vi "DNP3_Outstation_Main.vi"() -> ()   [LabVIEW 2016, in "DNP3_Outstation_Template.lvlib"]
uses:
  DNP3_Outstation_Template.lvlib
panel:
  out "STOP IND":bool
  out "RESET OS IND":bool
  out "ENABLE OS IND":bool=TRUE
  in  "STOP":bool
  out "MS POLLING? IND":bool=TRUE
  in  "OS Presets":T1(tab)
  in  "Network Settings 1":T2={"port (20000)"=18000, "Master IP"="48.26.87.212", "Master Address"=12345, "Outstation Address "=54321, " update rate"=50}
  in  "DNP3 DataMap 1":T3={"Binary Output Points"=1, "Binary Input Points"=0, "Analog Output Points"=7, "Analog Input Points"=6}
  in  "Settings Cluster":T4={"Default Variation:Analog Input Event (OBJ32)"=1, "Default Variation:Analog Input (OBJ30)"=1, "Default Variation:Binary Input (OBJ01)"=1, "Default Variation:Analog Output (OBJ40)"=4, "Default Variation:Binary Output Event (OBJ11)"=1, "Default Variation:Binary Output (OBJ10)"=1, "Default Variation:Analog Output Event (OBJ42)"=8, "Unsolicited Response Allowed"=FALSE, "Control:Select Timeout (ms)"=0, "Misc:Appl Confirmation Timeout"=0} {"Default Variation:Analog Output Event (OBJ42)" items=["32-bit without Time"=1, "16-bit without Time"=2, "32-bit with Time"=3, "16-bit with Time"=4, "Single-prec without Time"=5, "Double-prec without Time"=6, "Single-prec with Time"=7, "Double-prec with Time"=8]; "Default Variation:Binary Output (OBJ10)" items=["Packed Format"=1, "Output Status with Flags"=2]; "Default Variation:Binary Output Event (OBJ11)" items=["Status without Time"=1, "Status with Time"=2]; "Default Variation:Analog Output (OBJ40)" items=["32-bit with Flag"=1, "16-bit with Flag"=2, "Single-prec with Flag"=3, "Double-prec with Flag"=4]; "Default Variation:Binary Input (OBJ01)" items=["Packed Format"=1, "With Flags"=2]; "Default Variation:Analog Input (OBJ30)" items=["32-bit with Flag"=1, "16-bit with Flag"=2, "32-bit without Flag"=3, "16-bit without Flag"=4, "Single-prec with Flag"=5, "Double-prec with Flag"=6]; "Default Variation:Analog Input Event (OBJ32)" items=["32-bit without Time"=1, "16-bit without Time"=2, "32-bit with Time"=3, "16-bit with Time"=4, "Single-prec without Time"=5, "Double-prec without Time"=6, "Single-prec with Time"=7, "Double-prec with Time"=8]}
  in  "Network Settings 2":T2
  in  "DNP3 DataMap 2":T3
  in  "Settings Cluster 2":T4={"Default Variation:Analog Input Event (OBJ32)"=1, "Default Variation:Analog Input (OBJ30)"=1, "Default Variation:Binary Input (OBJ01)"=1, "Default Variation:Analog Output (OBJ40)"=1, "Default Variation:Binary Output Event (OBJ11)"=1, "Default Variation:Binary Output (OBJ10)"=1, "Default Variation:Analog Output Event (OBJ42)"=1, "Unsolicited Response Allowed"=FALSE, "Control:Select Timeout (ms)"=0, "Misc:Appl Confirmation Timeout"=0} {"Default Variation:Analog Output Event (OBJ42)" items=["32-bit without Time"=1, "16-bit without Time"=2, "32-bit with Time"=3, "16-bit with Time"=4, "Single-prec without Time"=5, "Double-prec without Time"=6, "Single-prec with Time"=7, "Double-prec with Time"=8]; "Default Variation:Binary Output (OBJ10)" items=["Packed Format"=1, "Output Status with Flags"=2]; "Default Variation:Binary Output Event (OBJ11)" items=["Status without Time"=1, "Status with Time"=2]; "Default Variation:Analog Output (OBJ40)" items=["32-bit with Flag"=1, "16-bit with Flag"=2, "Single-prec with Flag"=3, "Double-prec with Flag"=4]; "Default Variation:Binary Input (OBJ01)" items=["Packed Format"=1, "With Flags"=2]; "Default Variation:Analog Input (OBJ30)" items=["32-bit with Flag"=1, "16-bit with Flag"=2, "32-bit without Flag"=3, "16-bit without Flag"=4, "Single-prec with Flag"=5, "Double-prec with Flag"=6]; "Default Variation:Analog Input Event (OBJ32)" items=["32-bit without Time"=1, "16-bit without Time"=2, "32-bit with Time"=3, "16-bit with Time"=4, "Single-prec without Time"=5, "Double-prec without Time"=6, "Single-prec with Time"=7, "Double-prec with Time"=8]}
  in  "Network Settings 3":T2
  in  "DNP3 DataMap 3":T3
  in  "Settings Cluster 3":T4={"Default Variation:Analog Input Event (OBJ32)"=1, "Default Variation:Analog Input (OBJ30)"=1, "Default Variation:Binary Input (OBJ01)"=1, "Default Variation:Analog Output (OBJ40)"=1, "Default Variation:Binary Output Event (OBJ11)"=1, "Default Variation:Binary Output (OBJ10)"=1, "Default Variation:Analog Output Event (OBJ42)"=1, "Unsolicited Response Allowed"=FALSE, "Control:Select Timeout (ms)"=0, "Misc:Appl Confirmation Timeout"=0} {"Default Variation:Analog Output Event (OBJ42)" items=["32-bit without Time"=1, "16-bit without Time"=2, "32-bit with Time"=3, "16-bit with Time"=4, "Single-prec without Time"=5, "Double-prec without Time"=6, "Single-prec with Time"=7, "Double-prec with Time"=8]; "Default Variation:Binary Output (OBJ10)" items=["Packed Format"=1, "Output Status with Flags"=2]; "Default Variation:Binary Output Event (OBJ11)" items=["Status without Time"=1, "Status with Time"=2]; "Default Variation:Analog Output (OBJ40)" items=["32-bit with Flag"=1, "16-bit with Flag"=2, "Single-prec with Flag"=3, "Double-prec with Flag"=4]; "Default Variation:Binary Input (OBJ01)" items=["Packed Format"=1, "With Flags"=2]; "Default Variation:Analog Input (OBJ30)" items=["32-bit with Flag"=1, "16-bit with Flag"=2, "32-bit without Flag"=3, "16-bit without Flag"=4, "Single-prec with Flag"=5, "Double-prec with Flag"=6]; "Default Variation:Analog Input Event (OBJ32)" items=["32-bit without Time"=1, "16-bit without Time"=2, "32-bit with Time"=3, "16-bit with Time"=4, "Single-prec without Time"=5, "Double-prec without Time"=6, "Single-prec with Time"=7, "Double-prec with Time"=8]}
  out "Main VI Iterations":i32=2304
  out "OS SETTINGS CHANGED":bool
  in  "ENABLE OS":bool=TRUE
  in  "RESET OS":bool caption="Reset Outstation"
  out "OS SubVI Iterations":i16=1064
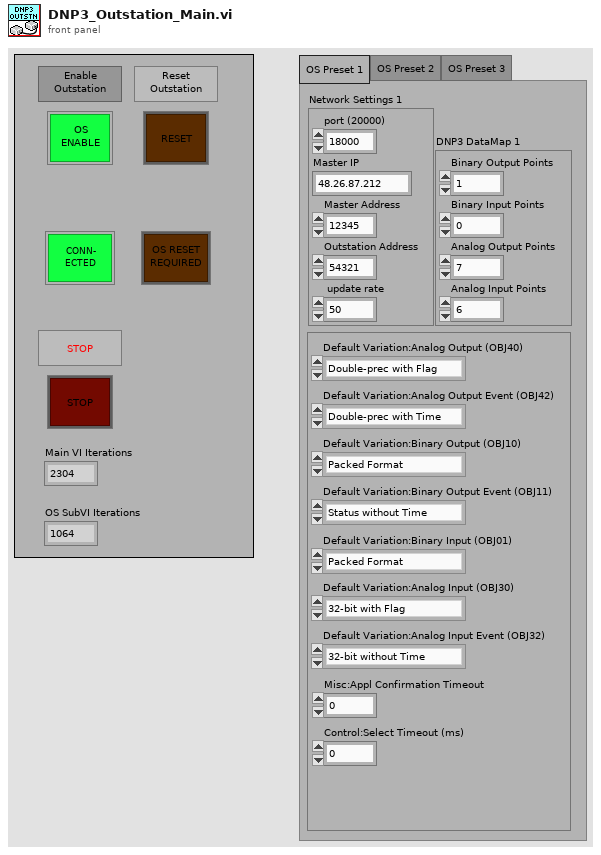
[diagram p1: front panel]
types:
  T1 = enum32{"OS Preset 1", "OS Preset 2", "OS Preset 3"}
  T2 = cluster{"port (20000)":u16, "Master IP":string, "Master Address":u16, "Outstation Address ":u16, " update rate":u32}
  T3 = cluster{"Binary Output Points":u16, "Binary Input Points":u16, "Analog Output Points":u16, "Analog Input Points":u16}
  T4 = cluster{"Default Variation:Analog Input Event (OBJ32)":u8, "Default Variation:Analog Input (OBJ30)":u8, "Default Variation:Binary Input (OBJ01)":u8, "Default Variation:Analog Output (OBJ40)":u8, "Default Variation:Binary Output Event (OBJ11)":u8, "Default Variation:Binary Output (OBJ10)":u8, "Default Variation:Analog Output Event (OBJ42)":u8, "Unsolicited Response Allowed":bool, "Control:Select Timeout (ms)":u32, "Misc:Appl Confirmation Timeout":u32}
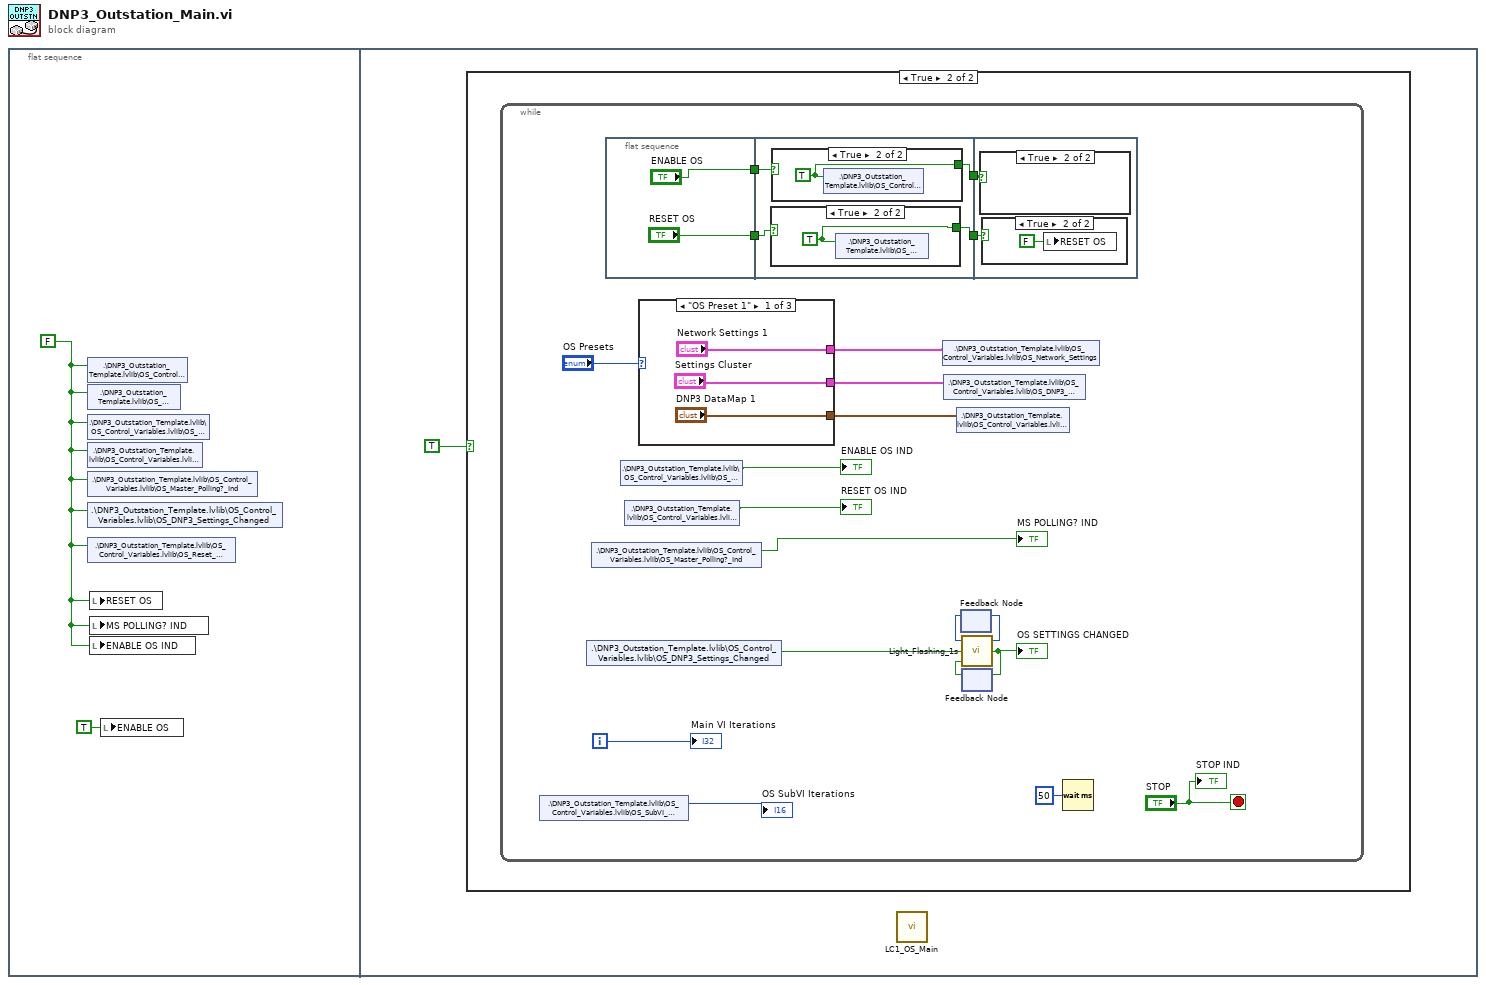
[diagram p0: block diagram]
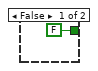
[diagram p3: hidden frame]
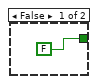
[diagram p4: hidden frame]
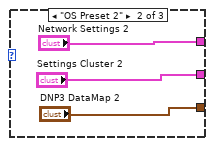
[diagram p7: hidden frame]
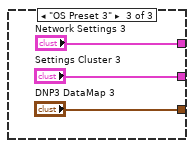
[diagram p8: hidden frame]
diagram:
  n1 = flat-sequence {
    frame #0 {
      w2 = FALSE ("LC1_MS_Enable")
      n2 = shared-variable ".\\DNP3_Outstation_Template.lvlib\\OS_Control_Variables.lvlib\\OS_Enable"(w2) -> ()  [unwired: 1 in, 1 out]
      n3 = shared-variable ".\\DNP3_Outstation_Template.lvlib\\OS_Control_Variables.lvlib\\OS_Reset"(w2) -> ()  [unwired: 1 in, 1 out]
      n4 = shared-variable ".\\DNP3_Outstation_Template.lvlib\\OS_Control_Variables.lvlib\\OS_Enable_Ind"(w2) -> ()  [unwired: 1 in, 1 out]
      n5 = shared-variable ".\\DNP3_Outstation_Template.lvlib\\OS_Control_Variables.lvlib\\OS_Reset_Ind"(w2) -> ()  [unwired: 1 in, 1 out]
      n6 = shared-variable ".\\DNP3_Outstation_Template.lvlib\\OS_Control_Variables.lvlib\\OS_Master_Polling?_Ind"(w2) -> ()  [unwired: 1 in, 1 out]
      n7 = shared-variable ".\\DNP3_Outstation_Template.lvlib\\OS_Control_Variables.lvlib\\OS_DNP3_Settings_Changed"(w2) -> ()  [unwired: 1 in, 1 out]
      n8 = shared-variable ".\\DNP3_Outstation_Template.lvlib\\OS_Control_Variables.lvlib\\OS_Reset_Succesful"(w2) -> ()  [unwired: 1 in, 1 out]
      n9 = local write "RESET OS"(w2) -> ()
      n10 = local write "MS POLLING? IND"(w2) -> ()
      n11 = local write "ENABLE OS IND"(w2) -> ()
      n12 = local write "ENABLE OS"(TRUE ("ENABLE OS")) -> ()
    }
    frame #1 {
      n13 = case shown="True" TRUE {
        frame False {
        }
        frame True {
          n14 = while {
            i -> [w20]
            stop <- "STOP" stop-if-true
            n15 = shared-variable ".\\DNP3_Outstation_Template.lvlib\\OS_Control_Variables.lvlib\\OS_SubVI_Iterations"() -> (→"OS SubVI Iterations":i32)  [unwired: 1 in, 1 out]
            n16 = shared-variable ".\\DNP3_Outstation_Template.lvlib\\OS_Control_Variables.lvlib\\OS_DNP3_Settings_Changed"() -> (w9:bool)  [unwired: 1 in, 1 out]
            n17 = shared-variable ".\\DNP3_Outstation_Template.lvlib\\OS_Control_Variables.lvlib\\OS_Master_Polling?_Ind"() -> (→"MS POLLING? IND":bool)  [unwired: 1 in, 1 out]
            n18 = flat-sequence {
              tunnel: ["ENABLE OS"] -> w19
              tunnel: ["RESET OS"] -> w18
              tunnel: w19 -> [w29]
              tunnel: w18 -> [w28]
              tunnel: [w27] -> w17
              tunnel: [w26] -> w16
              tunnel: w17 -> [w35]
              tunnel: w16 -> [w34]
              frame #0 {
              }
              frame #1 {
                n19 = case shown="True" w28 {
                  tunnel: [FALSE ("LC1_OS_Reset") w31] -> w26
                  frame False {
                  }
                  frame True {
                    w31 = TRUE ("LC1_OS_Reset")
                    n20 = shared-variable ".\\DNP3_Outstation_Template.lvlib\\OS_Control_Variables.lvlib\\OS_Reset"(w31) -> ()  [unwired: 1 in, 1 out]
                  }
                }
                n21 = case shown="True" w29 {
                  tunnel: [FALSE ("LC1_OS_Enable") w33] -> w27
                  frame False {
                  }
                  frame True {
                    w33 = TRUE ("LC1_OS_Enable")
                    n22 = shared-variable ".\\DNP3_Outstation_Template.lvlib\\OS_Control_Variables.lvlib\\OS_Enable"(w33) -> ()  [unwired: 1 in, 1 out]
                  }
                }
              }
              frame #2 {
                n23 = case shown="True" w35 {
                  frame False {
                  }
                  frame True {
                  }
                }
                n24 = case shown="True" w34 {
                  frame False {
                  }
                  frame True {
                    n25 = local write "RESET OS"(FALSE ("RESET OS")) -> ()
                  }
                }
              }
            }
            n26 = shared-variable ".\\DNP3_Outstation_Template.lvlib\\OS_Control_Variables.lvlib\\OS_Enable_Ind"() -> (→"ENABLE OS IND":bool)  [unwired: 1 in, 1 out]
            n27 = shared-variable ".\\DNP3_Outstation_Template.lvlib\\OS_Control_Variables.lvlib\\OS_Reset_Ind"() -> (→"RESET OS IND":bool)  [unwired: 1 in, 1 out]
            n28 = case shown="\"OS Preset 1\"" "OS Presets" {
              tunnel: ["Network Settings 1" "Network Settings 2" "Network Settings 3"] -> w6
              tunnel: ["Settings Cluster" "Settings Cluster 2" "Settings Cluster 3"] -> w5
              tunnel: ["DNP3 DataMap 1" "DNP3 DataMap 2" "DNP3 DataMap 3"] -> w4
              frame "OS Preset 1" {
              }
              frame "OS Preset 2" {
              }
              frame "OS Preset 3" {
              }
            }
            n29 = shared-variable ".\\DNP3_Outstation_Template.lvlib\\OS_Control_Variables.lvlib\\OS_Network_Settings"(w6) -> ()  [unwired: 1 in, 1 out]
            n30 = shared-variable ".\\DNP3_Outstation_Template.lvlib\\OS_Control_Variables.lvlib\\OS_DNP3_Settings"(w5) -> ()  [unwired: 1 in, 1 out]
            n31 = shared-variable ".\\DNP3_Outstation_Template.lvlib\\OS_Control_Variables.lvlib\\OS_DataMap"(w4) -> ()  [unwired: 1 in, 1 out]
            n32 = feedback #1() -> (w10:i32)  [unwired: 1 in]
            n33 = feedback #2() -> (w8:bool)  [unwired: 1 in]
            n34 = call "Light_Flashing_1s.vi"("Boolean 3"=w8, "Boolean"=w9, "Numeric 2"=w10) -> ("Boolean 2"=w12:bool, "Numeric"=w11:i32)  [unwired: 1 in]
            "OS SETTINGS CHANGED" <- w12
            n35 = feedback-in #1(w11) -> ()
            n36 = feedback-in #2(w12) -> ()
            n37 = Wait (ms)(milliseconds to wait=u32 50) -> ()  [unwired: 1 out]
            "STOP IND" <- "STOP"
            "Main VI Iterations" <- w20
          }
        }
      }
      n38 = call "LC1_OS_Main.vi"() -> ()  [unwired: 12 in]
    }
  }
